vi "SwerveModifyDriveCommand.vi"(0 "Raw Drive Command (ul)":dbl, 1 "Flip Drive Command":bool, 2 "Azimuth Error (deg)":dbl) -> (4 "Modified Drive Command (ul)":dbl format="%.3f")   [LabVIEW 2020]
doc: "This VI modifies the drive motor commands based on data from the azimuth controllers. It handles \"flipping\" the drive direction to minimize azimuthal travel and supresses the drive command when the module is pointed in the wrong direction."
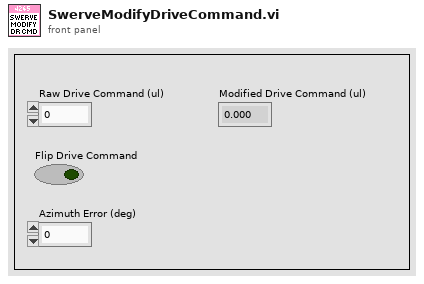
[diagram p1: front panel]
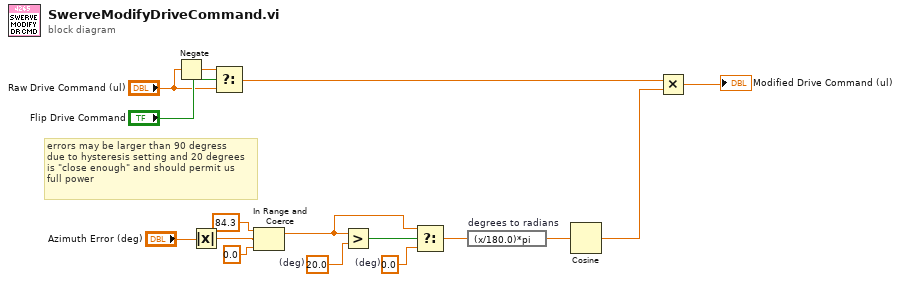
[diagram p0: block diagram]
diagram:
  w10 = 0.0  # (deg)
  w8 = 20.0  # (deg)
  # "errors may be larger than 90 degress\ndue to hysteresis setting and 20 degrees\nis \"close enough\" and should permit us\nfull power"
  n1 = Negate(x="Raw Drive Command (ul)") -> (-x=w4:dbl)
  n2 = Absolute Value(x="Azimuth Error (deg)") -> (abs(x)=w13:dbl)
  n3 = Select(t=w4, s="Flip Drive Command", f="Raw Drive Command (ul)") -> (s? t:f=w6:dbl)
  n4 = In Range and Coerce(upper limit=84.3, x=w13, lower limit=0.0) -> (coerced(x)=w9:dbl)  [unwired: 1 out]
  n5 = Greater?(x=w9, y=w8) -> (0:w11:bool)
  n6 = Select(t=w9, s=w11, f=w10) -> (s? t:f=w7:dbl)
  n7 = expression code="(x/180.0)*pi" "degrees to radians"(w7) -> (w12:dbl)
  n8 = Cosine(x=w12) -> (cos(x)=w1:dbl)
  n9 = Multiply(x=w6, y=w1) -> (x*y=→"Modified Drive Command (ul)":dbl)
